vi "Stop Heat.vi"(2 "IsFinished":bool, 8 "error in (no error)":errorcluster, 11 "Direct Oven in":refnum<class "Direct Oven.lvclass">) -> (0 "error out":errorcluster, 3 "Direct Oven out":refnum<class "Direct Oven.lvclass">)   [LabVIEW 2024, in "Oven Actor.lvlib" / "Direct Oven.lvclass"]
uses:
  Direct Oven.lvclass
  Direct Oven.lvclass/Direct Oven.ctl
  Oven Actor/Oven Actor.lvclass
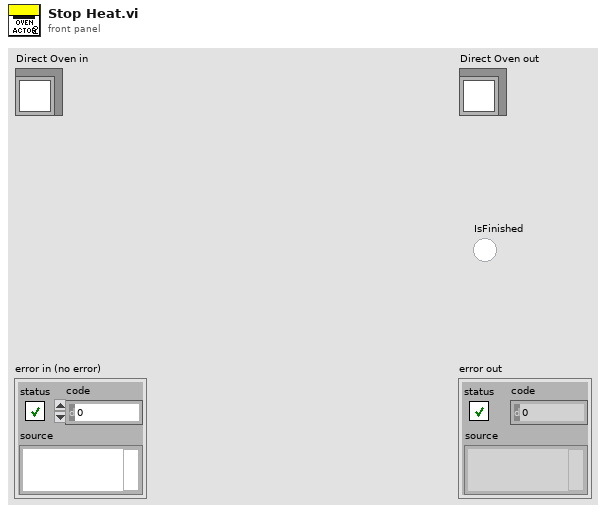
[diagram p1: front panel]
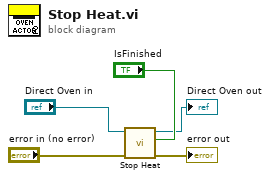
[diagram p0: block diagram]
diagram:
  n1 = call-parent "Stop Heat.vi"("IsFinished"="IsFinished", "error in (no error)"="error in (no error)", "Oven Actor in"="Direct Oven in") -> ("error out"=→"error out":errorcluster, "Oven Actor out"=→"Direct Oven out":refnum<class "Direct Oven.lvclass">)  [unwired: 7 in]
